vi "4461 - AI Read Data.vi"(8 "error in (no error)":errorcluster, 9 "sampling info":cluster{"Fs":dbl, "#s":dbl}={"Fs"=1000.0, "#s"=1000.0} {"Fs" format="%.2p"}, 11 "AI task":refnum<k21>[](array[refnum])=["", ""]) -> (0 "error out":errorcluster, 3 "Input Signals":waveform(dbl)[](array[waveform]))   [LabVIEW 2016, in "Instrument.Lockin.lvclass"]
uses:
  Instrument.Lockin.lvclass
  <vilib>/DAQmx/read.llb/DAQmx Read (Analog 1D Wfm NChan NSamp).vi
  <vilib>/DAQmx/miscellaneous.llb/DAQmx Fill In Error Info.vi
  <resource>/objmgr/daqmx.rc
panel:
  out "AvailSampPerChan 4":u32
  out "AvailSampPerChan 3":u32
  out "AvailSampPerChan 2":u32
  out "AvailSampPerChan 1":u32
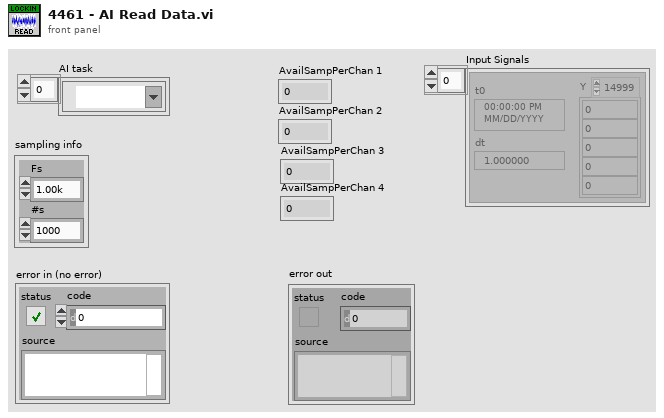
[diagram p1: front panel]
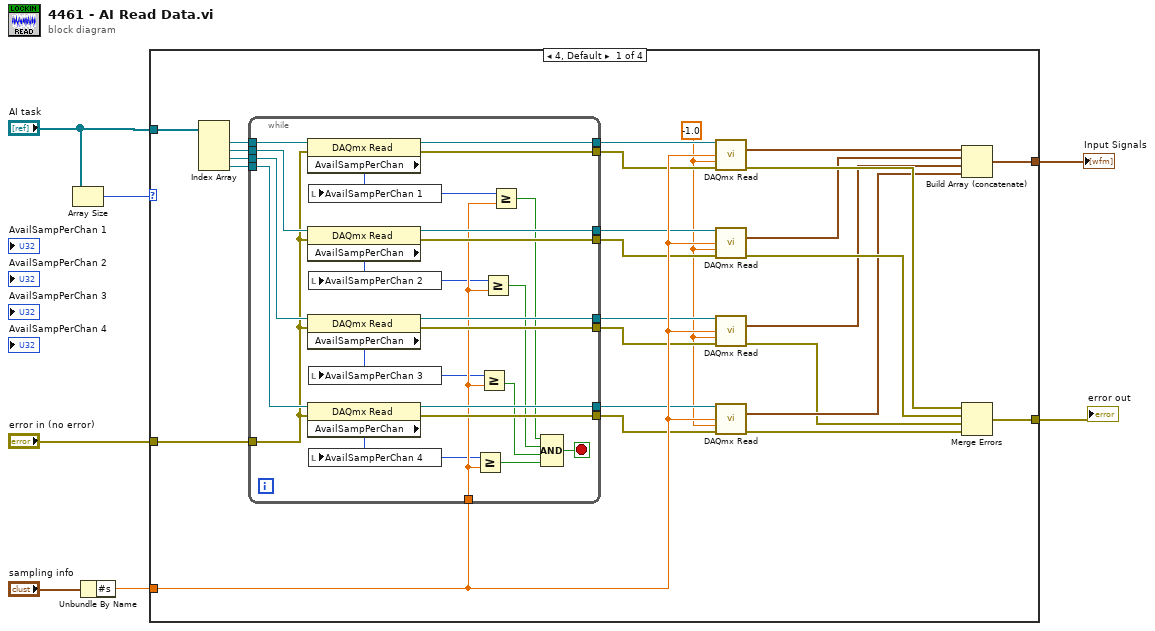
[diagram p0: block diagram]
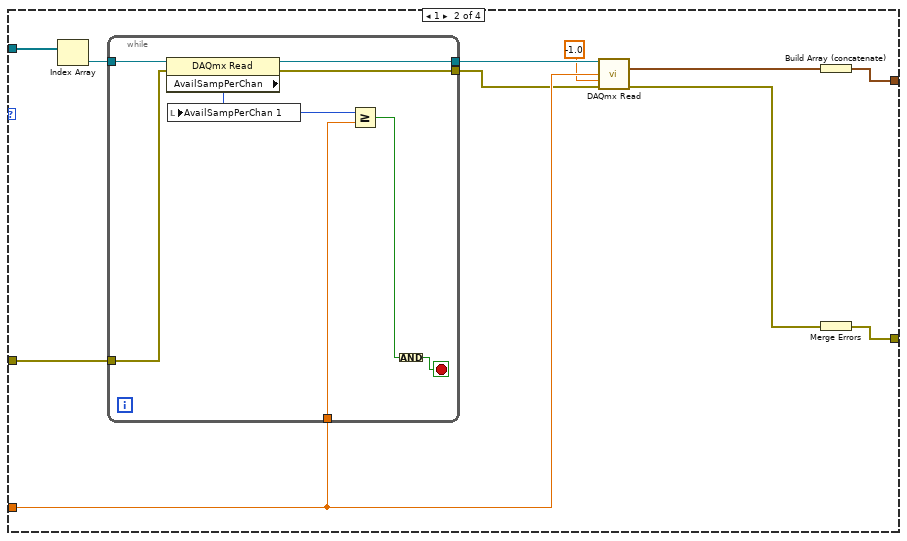
[diagram p2: hidden frame]
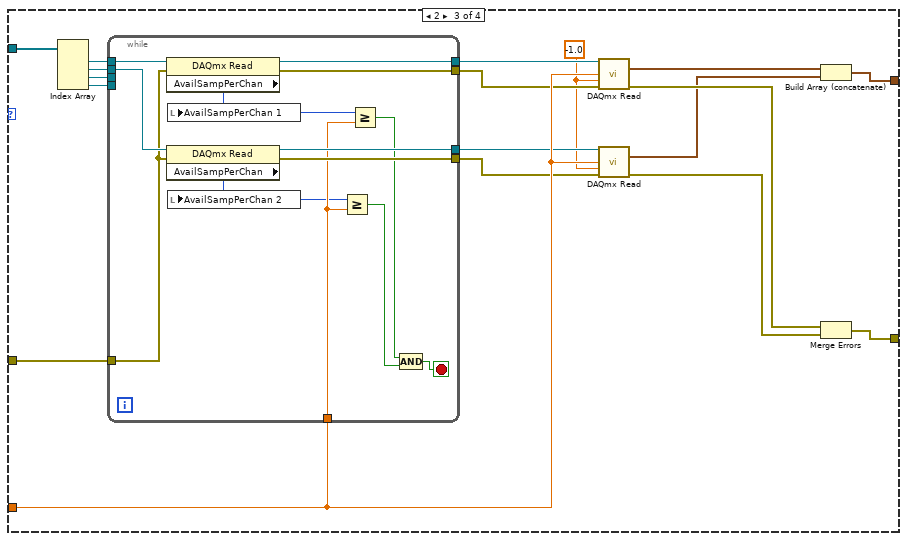
[diagram p3: hidden frame]
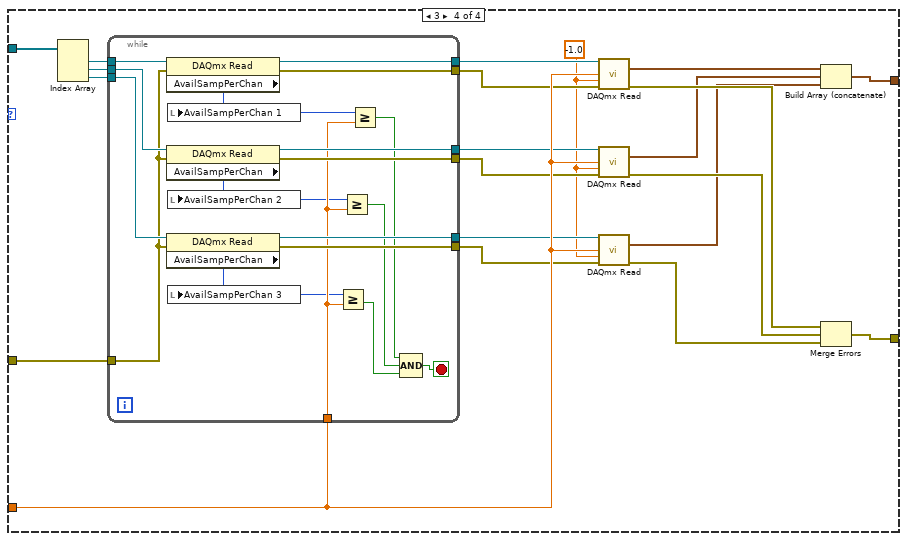
[diagram p4: hidden frame]
diagram:
  n1 = Array Size(array="AI task") -> (size(s)=w3:i32)
  n2 = Unbundle By Name("sampling info") -> ("#s"=w2:dbl)
  n3 = case shown="4, Default" w3 {
    tunnel: "AI task" -> [w33 w67 w93 w127]
    tunnel: [w32 w66 w92 w126] -> w6
    tunnel: "error in (no error)" -> [w31 w65 w91 w125]
    tunnel: [w29 w63 w89 w123] -> w4
    tunnel: w2 -> [w26 w62 w87 w121]
    frame 4, Default {
      w9 = -1.0 ("timeout")
      n4 = Index Array(array=w33) -> (element #1=w18:refnum<k21>, element #2=w19:refnum<k21>, element #3=w20:refnum<k21>, element #4=w21:refnum<k21>)  [unwired: 4 in]
      n5 = while {
        tunnel: w21 -> [w56]
        tunnel: w20 -> [w55]
        tunnel: w19 -> [w54]
        tunnel: w18 -> [w53]
        tunnel: [w52] -> w17
        tunnel: [w51] -> w16
        tunnel: [w50] -> w15
        tunnel: [w49] -> w14
        tunnel: w31 -> [w44]
        tunnel: [w48] -> w13
        tunnel: [w47] -> w12
        tunnel: [w46] -> w11
        tunnel: [w45] -> w10
        tunnel: w26 -> [w42]
        stop <- w34 stop-if-true
        n6 = property class="DAQmx Read"(reference=w53, error in=w44) -> (reference out=w52:refnum<k21>, error out=w48:errorcluster, "AvailSampPerChan"=w43:u32)
        n7 = property class="DAQmx Read"(reference=w54, error in=w44) -> (reference out=w51:refnum<k21>, error out=w47:errorcluster, "AvailSampPerChan"=w39:u32)
        n8 = property class="DAQmx Read"(reference=w55, error in=w44) -> (reference out=w50:refnum<k21>, error out=w46:errorcluster, "AvailSampPerChan"=w40:u32)
        n9 = property class="DAQmx Read"(reference=w56, error in=w44) -> (reference out=w49:refnum<k21>, error out=w45:errorcluster, "AvailSampPerChan"=w41:u32)
        n10 = local write "AvailSampPerChan 1"(w43) -> ()
        n11 = local write "AvailSampPerChan 2"(w39) -> ()
        n12 = local write "AvailSampPerChan 3"(w40) -> ()
        n13 = local write "AvailSampPerChan 4"(w41) -> ()
        n14 = Greater Or Equal?(x=w41, y=w42) -> (x >= y?=w38:bool)
        n15 = Greater Or Equal?(x=w40, y=w42) -> (x >= y?=w37:bool)
        n16 = Greater Or Equal?(x=w39, y=w42) -> (x >= y?=w36:bool)
        n17 = Greater Or Equal?(x=w43, y=w42) -> (x >= y?=w35:bool)
        n18 = Compound Arithmetic op=AND(w35, w36, w37, w38) -> (w34:bool)
      }
      n19 = call-poly <vilib>:"DAQmx Read.vi"("task/channels in"=w17, "number of samples per channel"=w26, "timeout"=w9, "error in"=w13) -> ("data"=w22:waveform(dbl)[], "error out"=w30:errorcluster)  [unwired: 9 in, 1 out]
      n20 = call-poly <vilib>:"DAQmx Read.vi"("task/channels in"=w16, "number of samples per channel"=w26, "timeout"=w9, "error in"=w12) -> ("data"=w23:waveform(dbl)[], "error out"=w28:errorcluster)  [unwired: 9 in, 1 out]
      n21 = call-poly <vilib>:"DAQmx Read.vi"("task/channels in"=w15, "number of samples per channel"=w26, "timeout"=w9, "error in"=w11) -> ("data"=w24:waveform(dbl)[], "error out"=w8:errorcluster)  [unwired: 9 in, 1 out]
      n22 = call-poly <vilib>:"DAQmx Read.vi"("task/channels in"=w14, "number of samples per channel"=w26, "timeout"=w9, "error in"=w10) -> ("data"=w25:waveform(dbl)[], "error out"=w27:errorcluster)  [unwired: 9 in, 1 out]
      n23 = Build Array (concatenate)(w22, w23, w24, w25) -> (w32:waveform(dbl)[])
      n24 = Merge Errors(w30, w28, w8, w27) -> (w29:errorcluster)
    }
    frame 1 {
      n25 = Index Array(array=w67) -> (element=w60:refnum<k21>)  [unwired: 1 in]
      n26 = while {
        tunnel: w60 -> [w75]
        tunnel: [w74] -> w59
        tunnel: w65 -> [w72]
        tunnel: [w73] -> w58
        tunnel: w62 -> [w70]
        stop <- w68 stop-if-true
        n27 = property class="DAQmx Read"(reference=w75, error in=w72) -> (reference out=w74:refnum<k21>, error out=w73:errorcluster, "AvailSampPerChan"=w71:u32)
        n28 = local write "AvailSampPerChan 1"(w71) -> ()
        n29 = Greater Or Equal?(x=w71, y=w70) -> (x >= y?=w69:bool)
        n30 = Compound Arithmetic op=AND(w69) -> (w68:bool)
      }
      n31 = call-poly <vilib>:"DAQmx Read.vi"("task/channels in"=w59, "number of samples per channel"=w62, "timeout"=-1.0, "error in"=w58) -> ("data"=w61:waveform(dbl)[], "error out"=w64:errorcluster)  [unwired: 9 in, 1 out]
      n32 = Build Array (concatenate)(w61) -> (w66:waveform(dbl)[])
      n33 = Merge Errors(w64) -> (w63:errorcluster)
    }
    frame 2 {
      w76 = -1.0 ("timeout")
      n34 = Index Array(array=w93) -> (element #1=w81:refnum<k21>, element #2=w82:refnum<k21>, element #3=w83:refnum<k21>, element #4=w84:refnum<k21>)  [unwired: 4 in]
      n35 = while {
        tunnel: w84 -> [_]
        tunnel: w83 -> [_]
        tunnel: w82 -> [w106]
        tunnel: w81 -> [w105]
        tunnel: [w104] -> w80
        tunnel: [w103] -> w79
        tunnel: w91 -> [w100]
        tunnel: [w102] -> w78
        tunnel: [w101] -> w77
        tunnel: w87 -> [w98]
        stop <- w94 stop-if-true
        n36 = property class="DAQmx Read"(reference=w105, error in=w100) -> (reference out=w104:refnum<k21>, error out=w102:errorcluster, "AvailSampPerChan"=w99:u32)
        n37 = property class="DAQmx Read"(reference=w106, error in=w100) -> (reference out=w103:refnum<k21>, error out=w101:errorcluster, "AvailSampPerChan"=w97:u32)
        n38 = local write "AvailSampPerChan 1"(w99) -> ()
        n39 = local write "AvailSampPerChan 2"(w97) -> ()
        n40 = Greater Or Equal?(x=w97, y=w98) -> (x >= y?=w96:bool)
        n41 = Greater Or Equal?(x=w99, y=w98) -> (x >= y?=w95:bool)
        n42 = Compound Arithmetic op=AND(w95, w96) -> (w94:bool)
      }
      n43 = call-poly <vilib>:"DAQmx Read.vi"("task/channels in"=w80, "number of samples per channel"=w87, "timeout"=w76, "error in"=w78) -> ("data"=w85:waveform(dbl)[], "error out"=w90:errorcluster)  [unwired: 9 in, 1 out]
      n44 = call-poly <vilib>:"DAQmx Read.vi"("task/channels in"=w79, "number of samples per channel"=w87, "timeout"=w76, "error in"=w77) -> ("data"=w86:waveform(dbl)[], "error out"=w88:errorcluster)  [unwired: 9 in, 1 out]
      n45 = Build Array (concatenate)(w85, w86) -> (w92:waveform(dbl)[])
      n46 = Merge Errors(w90, w88) -> (w89:errorcluster)
    }
    frame 3 {
      w108 = -1.0 ("timeout")
      n47 = Index Array(array=w127) -> (element #1=w115:refnum<k21>, element #2=w116:refnum<k21>, element #3=w117:refnum<k21>)  [unwired: 3 in]
      n48 = while {
        tunnel: w117 -> [w145]
        tunnel: w116 -> [w144]
        tunnel: w115 -> [w143]
        tunnel: [w142] -> w114
        tunnel: [w141] -> w113
        tunnel: [w140] -> w112
        tunnel: w125 -> [w136]
        tunnel: [w139] -> w111
        tunnel: [w138] -> w110
        tunnel: [w137] -> w109
        tunnel: w121 -> [w134]
        stop <- w128 stop-if-true
        n49 = property class="DAQmx Read"(reference=w143, error in=w136) -> (reference out=w142:refnum<k21>, error out=w139:errorcluster, "AvailSampPerChan"=w135:u32)
        n50 = property class="DAQmx Read"(reference=w144, error in=w136) -> (reference out=w141:refnum<k21>, error out=w138:errorcluster, "AvailSampPerChan"=w132:u32)
        n51 = property class="DAQmx Read"(reference=w145, error in=w136) -> (reference out=w140:refnum<k21>, error out=w137:errorcluster, "AvailSampPerChan"=w133:u32)
        n52 = local write "AvailSampPerChan 1"(w135) -> ()
        n53 = local write "AvailSampPerChan 2"(w132) -> ()
        n54 = local write "AvailSampPerChan 3"(w133) -> ()
        n55 = Greater Or Equal?(x=w133, y=w134) -> (x >= y?=w131:bool)
        n56 = Greater Or Equal?(x=w132, y=w134) -> (x >= y?=w130:bool)
        n57 = Greater Or Equal?(x=w135, y=w134) -> (x >= y?=w129:bool)
        n58 = Compound Arithmetic op=AND(w129, w130, w131) -> (w128:bool)
      }
      n59 = call-poly <vilib>:"DAQmx Read.vi"("task/channels in"=w114, "number of samples per channel"=w121, "timeout"=w108, "error in"=w111) -> ("data"=w118:waveform(dbl)[], "error out"=w124:errorcluster)  [unwired: 9 in, 1 out]
      n60 = call-poly <vilib>:"DAQmx Read.vi"("task/channels in"=w113, "number of samples per channel"=w121, "timeout"=w108, "error in"=w110) -> ("data"=w119:waveform(dbl)[], "error out"=w122:errorcluster)  [unwired: 9 in, 1 out]
      n61 = call-poly <vilib>:"DAQmx Read.vi"("task/channels in"=w112, "number of samples per channel"=w121, "timeout"=w108, "error in"=w109) -> ("data"=w120:waveform(dbl)[], "error out"=w107:errorcluster)  [unwired: 9 in, 1 out]
      n62 = Build Array (concatenate)(w118, w119, w120) -> (w126:waveform(dbl)[])
      n63 = Merge Errors(w124, w122, w107) -> (w123:errorcluster)
    }
  }
  "Input Signals" <- w6
  "error out" <- w4
